vi "GL_Range_to_Delta.vi"(5 "Input":string, 7 "TUnit":string="C", 8 "Range":string) -> (1 "Unit":string, 2 "delta":dbl, 4 "Fmt":string)   [LabVIEW 2017]
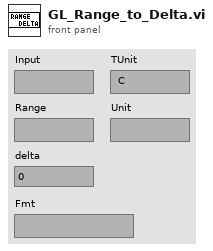
[diagram p1: front panel]
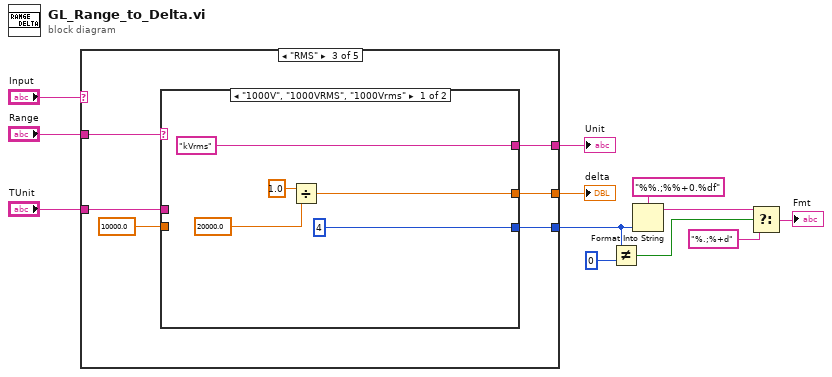
[diagram p0: block diagram]
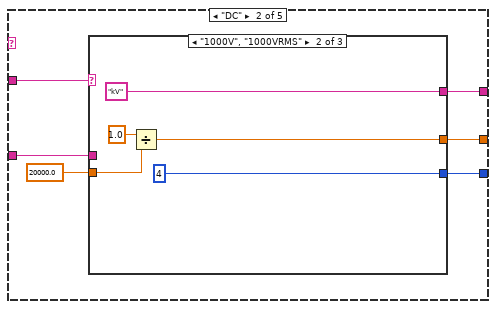
[diagram p3: hidden frame]
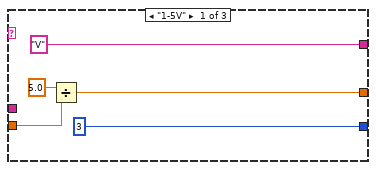
[diagram p4: hidden frame]
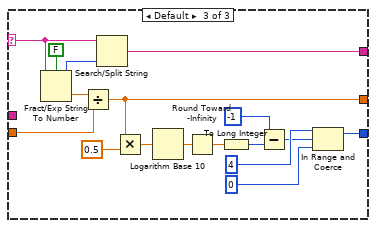
[diagram p5: hidden frame]
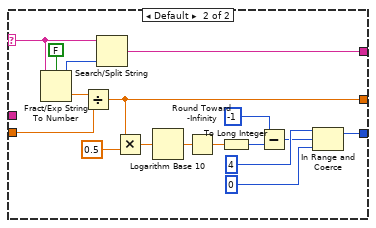
[diagram p6: hidden frame]
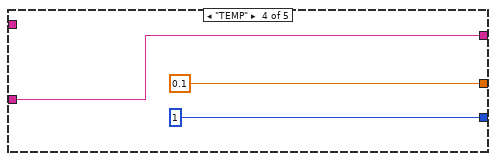
[diagram p7: hidden frame]
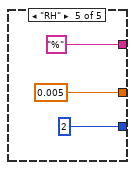
[diagram p8: hidden frame]
diagram:
  n1 = case shown="\"RMS\"" "Input" {
    tunnel: [_ w18 w51 0.1 0.005] -> w12
    tunnel: [_ w17 w50 w75 "%" ("TUnit")] -> w11
    tunnel: "TUnit" -> [_ w16 w49 w75 _]
    tunnel: [_ w15 w48 1 2] -> w4
    tunnel: "Range" -> [_ w13 w46 _ _]
    frame Default {
    }
    frame "DC" {
      n2 = case shown="\"1000V\", \"1000VRMS\"" w13 {
        selector: w13 -> [_ _ w30]
        tunnel: [w20 w25 w37] -> w18
        tunnel: ["V" ("Range") "kV" ("Range") w43] -> w17
        tunnel: w16 -> [_ _ _]
        tunnel: 20000.0 -> [w22 w27 w42]
        tunnel: [3 4 w31] -> w15
        frame "1-5V" {
          n3 = Divide(x=5.0, y=w22) -> (x/y=w20:dbl)
        }
        frame "1000V", "1000VRMS" {
          n4 = Divide(x=1.0, y=w27) -> (x/y=w25:dbl)
        }
        frame Default {
          n5 = Fract/Exp String To Number(use system decimal point (T)=FALSE, string=w30) -> (offset past number=w45:i32, number=w44:dbl)  [unwired: 2 out]
          n6 = Divide(x=w44, y=w42) -> (x/y=w37:dbl)
          n7 = Search/Split String(string=w30, offset (0)=w45) -> (match + rest of string=w43:string)  [unwired: 3 out]
          n8 = Multiply(x=w37, y=0.5) -> (x*y=w40:dbl)
          n9 = Logarithm Base 10(1:w40) -> (0:w39:dbl)
          n10 = Round Toward -Infinity(1:w39) -> (0:w38:dbl)
          n11 = To Long Integer(number=w38) -> (32bit integer=w35:i32)
          n12 = Subtract(x=-1, y=w35) -> (x-y=w32:i32)
          n13 = In Range and Coerce(upper limit=4, x=w32, lower limit=0) -> (coerced(x)=w31:i32)  [unwired: 1 out]
        }
      }
    }
    frame "RMS" {
      n14 = case shown="\"1000V\", \"1000VRMS\", \"1000Vrms\"" w46 {
        selector: w46 -> [_ w58]
        tunnel: [w54 w65] -> w51
        tunnel: ["kVrms" ("Range") w71] -> w50
        tunnel: w49 -> [_ _]
        tunnel: 10000.0 -> [_ w70]
        tunnel: [4 w59] -> w48
        frame "1000V", "1000VRMS", "1000Vrms" {
          n15 = Divide(x=1.0, y=20000.0) -> (x/y=w54:dbl)
        }
        frame Default {
          n16 = Fract/Exp String To Number(use system decimal point (T)=FALSE, string=w58) -> (offset past number=w73:i32, number=w72:dbl)  [unwired: 2 out]
          n17 = Divide(x=w72, y=w70) -> (x/y=w65:dbl)
          n18 = Search/Split String(string=w58, offset (0)=w73) -> (match + rest of string=w71:string)  [unwired: 3 out]
          n19 = Multiply(x=w65, y=0.5) -> (x*y=w68:dbl)
          n20 = Logarithm Base 10(1:w68) -> (0:w67:dbl)
          n21 = Round Toward -Infinity(1:w67) -> (0:w66:dbl)
          n22 = To Long Integer(number=w66) -> (32bit integer=w63:i32)
          n23 = Subtract(x=-1, y=w63) -> (x-y=w60:i32)
          n24 = In Range and Coerce(upper limit=4, x=w60, lower limit=0) -> (coerced(x)=w59:i32)  [unwired: 1 out]
        }
      }
    }
    frame "TEMP" {
    }
    frame "RH" {
    }
  }
  "delta" <- w12
  "Unit" <- w11
  n25 = Not Equal?(x=w4, y=0) -> (x != y?=w8:bool)
  n26 = Format Into String(format string="%%.;%%+0.%df", w4) -> (resulting string=w7:string)  [unwired: 2 in, 1 out]
  n27 = Select(t=w7, s=w8, f="%.;%+d" ("format string")) -> (s? t:f=→"Fmt":string)
